vi "自动保存XLS.vi"(0 "MCListbox引用句柄":refnum<vi>) -> ()   [LabVIEW 2014]
uses:
  <vilib>/Utility/file.llb/Write To Spreadsheet File (string).vi
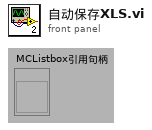
[diagram p1: front panel]
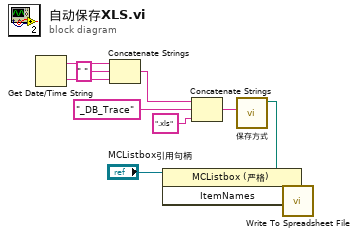
[diagram p0: block diagram]
diagram:
  n1 = Get Date/Time String() -> (date string=w3:string, time string=w4:string)  [unwired: 3 in]
  n2 = Concatenate Strings(w3, " " ("字符串"), w4) -> (w5:string)
  n3 = property on="属性节点" class="MCListbox (严格)"(reference="MCListbox引用句柄") -> ("ItemNames"=w2:string[][])  [unwired: 1 in, 2 out]
  n4 = Concatenate Strings(w5, "_DB_Trace" ("字符串"), ".xls" ("名称或相对路径")) -> (w8:string)
  n5 = call "保存方式.vi"("名称或相对路径"=w8) -> ("添加的路径"=w10:path)  [unwired: 10 in]
  n6 = call-poly <vilib>:"Write To Spreadsheet File.vi"("2D data"=w2, "file path (dialog if empty)"=w10) -> ()  [unwired: 6 in, 1 out]
